vi "Keyboard Input with Sensitivity Support.vi"(0 "error in (no error)":errorcluster, 1 "Speed step":dbl, 2 "Previous Control Cluster":T2 {"Yaw Speed" scale=-1.0..1.0; "Vertical Speed" scale=-1.0..1.0; "Pitch" scale=-1.0..1.0; "Roll" scale=-1.0..1.0}, 3 "device ID":refnum<k1>) -> (4 "Control Cluster":T3 {"Roll" scale=-1.0..1.0; "Pitch" scale=-1.0..1.0; "Vertical Speed" scale=-1.0..1.0; "Yaw Speed" scale=-1.0..1.0}, 5 "error out":errorcluster, 6 "Buttons control":T1)   [LabVIEW 2014]
uses:
  <vilib>/Utility/inputDevices.llb/keyboardAcquire.vi
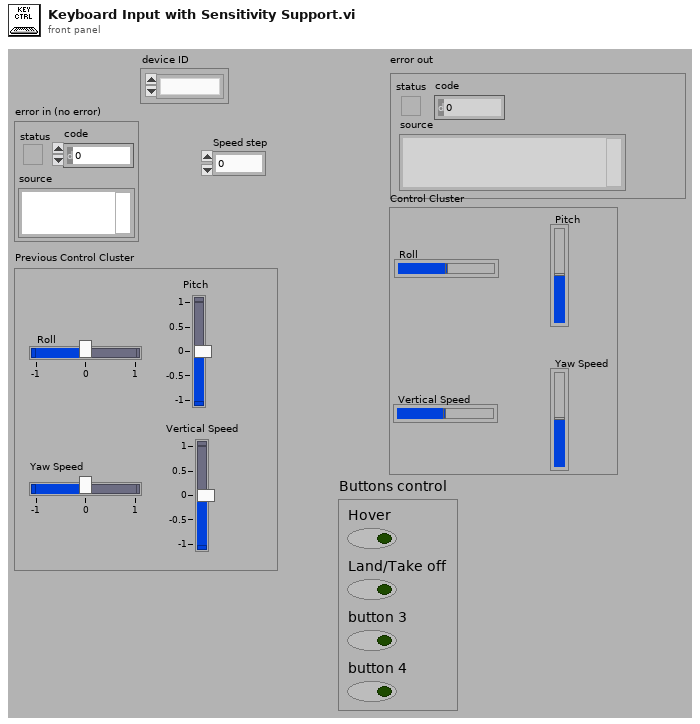
[diagram p1: front panel]
types:
  T1 = cluster{"Hover":bool, "Land/Take off":bool, "button 3":bool, "button 4":bool}
  T2 = cluster{"Roll":sgl, "Pitch":sgl, "Vertical Speed":sgl, "Yaw Speed":sgl}
  T3 = cluster{"Roll":dbl, "Pitch":dbl, "Vertical Speed":dbl, "Yaw Speed":dbl}
  T4 = enum16{"0", "1", "2", "3", "4", "5", "6", "7", "8", "9", "A", "B", "C", "D", "E", "F", "G", "H", "I", "J", "K", "L", "M", "N", "O", "P", "Q", "R", "S", "T", "U", "V", "W", "X", "Y", "Z", "F1", "F2", "F3", "F4", "F5", "F6", "F7", "F8", "F9", "F10", "F11", "F12", "F13", "F14", "F15", "ADD", "BACK", "BACKSLASH", "CAPITAL", "COMMA", "DECIMAL", "DELETE", "DIVIDE", "DOWN", "END", "EQUALS", "ESCAPE", "GRAVE (`)", "HOME", "INSERT", "LBRACKET", "LCONTROL", "LEFT", "L ALT", "LSHIFT", "LWIN", "MINUS", "MULTIPLY", "NEXT", "NUMLOCK", "NUMPAD_0", "NUMPAD_1", "NUMPAD_2", "NUMPAD_3", "NUMPAD_4", "NUMPAD_5", "NUMPAD_6", "NUMPAD_7", "NUMPAD_8", "NUMPAD_9", "PAUSE", "PERIOD", "PRIOR (PG UP)", "RBRACKET", "RCONTROL", "RETURN", "RIGHT", "R ALT", "RSHIFT", "RWIN", "SCROLL", "SEMICOLON", "SLASH", "SPACE", "SUBTRACT", "TAB", "UP", "ENTER (num pad)", "' (quote)"}[]
  T5 = enum16{"0", "1", "2", "3", "4", "5", "6", "7", "8", "9", "A", "B", "C", "D", "E", "F", "G", "H", "I", "J", "K", "L", "M", "N", "O", "P", "Q", "R", "S", "T", "U", "V", "W", "X", "Y", "Z", "F1", "F2", "F3", "F4", "F5", "F6", "F7", "F8", "F9", "F10", "F11", "F12", "F13", "F14", "F15", "ADD", "BACK", "BACKSLASH", "CAPITAL", "COMMA", "DECIMAL", "DELETE", "DIVIDE", "DOWN", "END", "EQUALS", "ESCAPE", "GRAVE (`)", "HOME", "INSERT", "LBRACKET", "LCONTROL", "LEFT", "L ALT", "LSHIFT", "LWIN", "MINUS", "MULTIPLY", "NEXT", "NUMLOCK", "NUMPAD_0", "NUMPAD_1", "NUMPAD_2", "NUMPAD_3", "NUMPAD_4", "NUMPAD_5", "NUMPAD_6", "NUMPAD_7", "NUMPAD_8", "NUMPAD_9", "PAUSE", "PERIOD", "PRIOR (PG UP)", "RBRACKET", "RCONTROL", "RETURN", "RIGHT", "R ALT", "RSHIFT", "RWIN", "SCROLL", "SEMICOLON", "SLASH", "SPACE", "SUBTRACT", "TAB", "UP", "ENTER (num pad)", "' (quote)"}
  T6 = cluster{dbl, dbl, "New Speed":dbl, "New Speed":dbl}
  T7 = cluster{dbl, "New Speed":dbl, "New Speed":dbl, dbl}
  T8 = cluster{"New Speed":dbl, dbl, "New Speed":dbl, dbl}
  T9 = cluster{dbl, "New Speed":dbl, dbl, "New Speed":dbl}
  T10 = cluster{"New Speed":dbl, dbl, dbl, "New Speed":dbl}
  T11 = cluster{"New Speed":dbl, "New Speed":dbl, dbl, dbl}
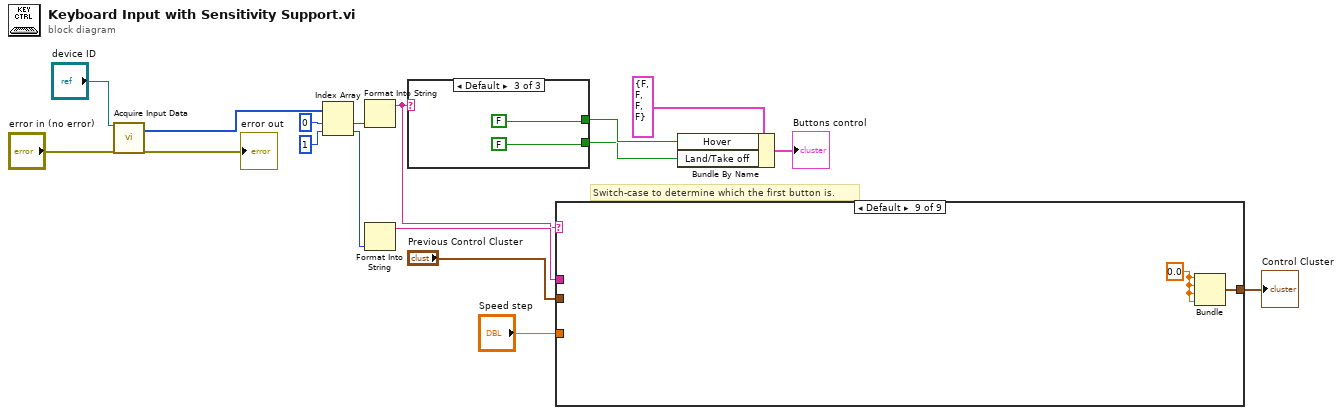
[diagram p0: block diagram]
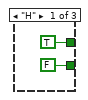
[diagram p2: hidden frame]
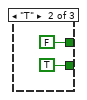
[diagram p3: hidden frame]
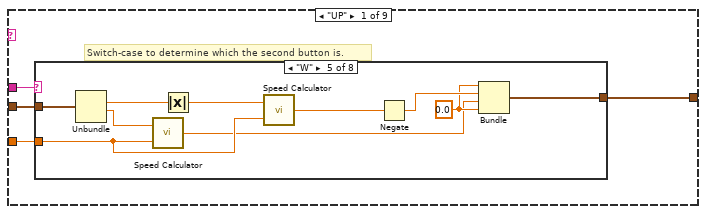
[diagram p4: hidden frame]
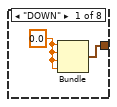
[diagram p5: hidden frame]
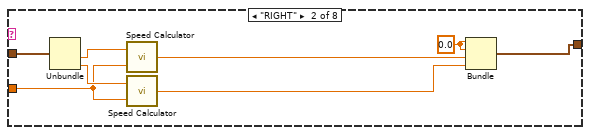
[diagram p6: hidden frame]
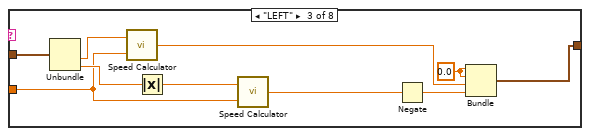
[diagram p7: hidden frame]
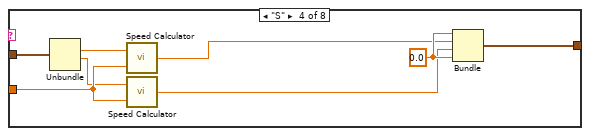
[diagram p8: hidden frame]
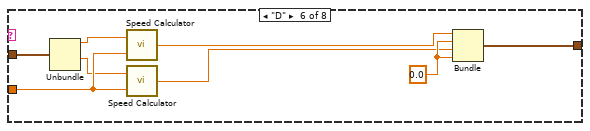
[diagram p9: hidden frame]
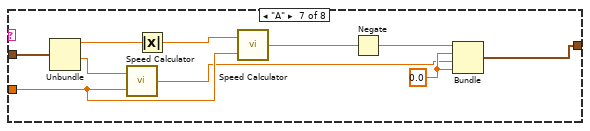
[diagram p10: hidden frame]
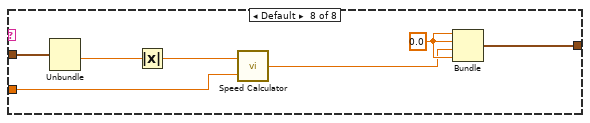
[diagram p11: hidden frame]
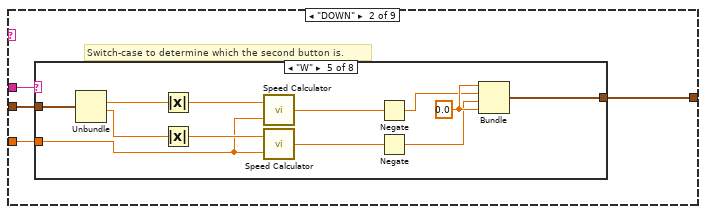
[diagram p12: hidden frame]
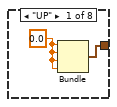
[diagram p13: hidden frame]
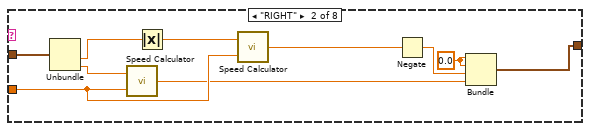
[diagram p14: hidden frame]
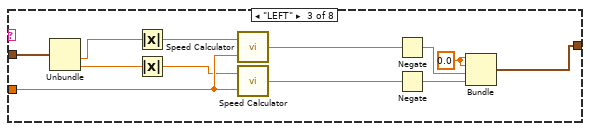
[diagram p15: hidden frame]
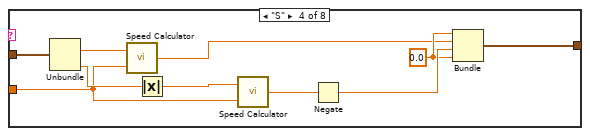
[diagram p16: hidden frame]
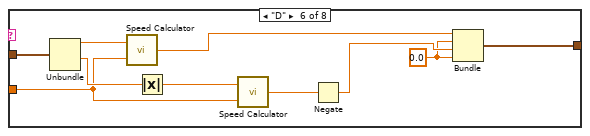
[diagram p17: hidden frame]
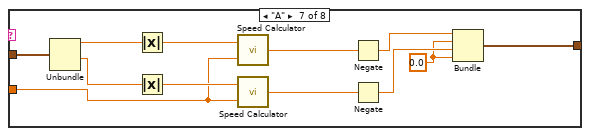
[diagram p18: hidden frame]
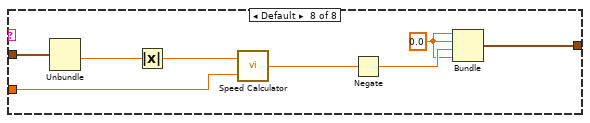
[diagram p19: hidden frame]
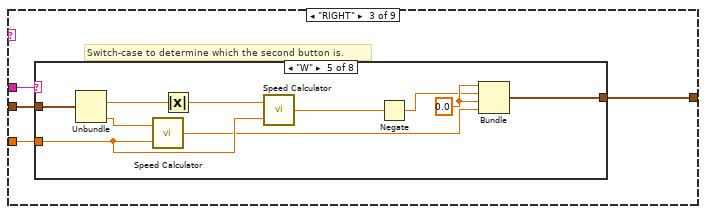
[diagram p20: hidden frame]
diagram:
  # "Switch-case to determine which the first button is."
  n1 = call-poly <vilib>:"Acquire Input Data.vi"("device ID"="device ID", "error in (no error)"="error in (no error)") -> ("keys pressed"=w12:T4, "error out"=→"error out":errorcluster)  [unwired: 15 in, 1 out]
  n2 = Index Array(array=w12, index #1=0, index #2=1) -> (element #1=w16:T5, element #2=w10:T5)
  n3 = Format Into String(w16) -> (resulting string=w5:string)  [unwired: 3 in, 1 out]
  n4 = Format Into String(w10) -> (resulting string=w9:string)  [unwired: 3 in, 1 out]
  n5 = case shown="Default" w5 {
    tunnel: [TRUE FALSE FALSE] -> w2
    tunnel: [FALSE TRUE FALSE] -> w1
    frame "H" {
    }
    frame "T" {
    }
    frame Default {
    }
  }
  n6 = case shown="Default" w5 {
    tunnel: w9 -> [w27 w93 w173 w240 w319 w385 w465 w531 _]
    tunnel: [w26 w92 w172 w238 w318 w384 w464 w530 w609] -> w7
    tunnel: "Speed step" -> [w25 w94 w174 w239 w320 w386 w466 w532 _]
    tunnel: "Previous Control Cluster" -> [w24 w91 w171 w237 w317 w383 w463 w529 _]
    frame "UP" {
      # "Switch-case to determine which the second button is."
      n7 = case shown="\"W\"" w27 {
        tunnel: [w28 w36 w47 w55 w65 w73 w83 w89] -> w26
        tunnel: w25 -> [_ w32 w41 w52 w59 w69 w78 w88]
        tunnel: w24 -> [_ w35 w44 w53 w62 w71 w80 w86]
        frame "DOWN" {
          w29 = 0.0
          n8 = Bundle(w29, w29, w29, w29) -> (w28:cluster{dbl, dbl, dbl, dbl})  [unwired: 1 in]
        }
        frame "RIGHT" {
          w37 = 0.0
          n9 = Unbundle(w35) -> ("Vertical Speed"=w30:sgl, "Yaw Speed"=w33:sgl)  [unwired: 2 out]
          n10 = call "Speed Calculator.vi"("Speed step"=w32, "Previous Speed"=w30) -> ("New Speed"=w34:dbl)
          n11 = call "Speed Calculator.vi"("Speed step"=w32, "Previous Speed"=w33) -> ("New Speed"=w31:dbl)
          n12 = Bundle(w37, w37, "New Speed"=w34, "New Speed"=w31) -> (w36:T6)  [unwired: 1 in]
        }
        frame "LEFT" {
          w45 = 0.0
          n13 = Unbundle(w44) -> ("Vertical Speed"=w40:sgl, "Yaw Speed"=w43:sgl)  [unwired: 2 out]
          n14 = call "Speed Calculator.vi"("Speed step"=w41, "Previous Speed"=w40) -> ("New Speed"=w39:dbl)
          n15 = Absolute Value(x=w43) -> (abs(x)=w42:sgl)
          n16 = call "Speed Calculator.vi"("Speed step"=w41, "Previous Speed"=w42) -> ("New Speed"=w38:dbl)
          n17 = Negate(x=w38) -> (-x=w46:dbl)
          n18 = Bundle(w45, w45, "New Speed"=w39, w46) -> (w47:cluster{dbl, dbl, "New Speed":dbl, dbl})  [unwired: 1 in]
        }
        frame "S" {
          w54 = 0.0
          n19 = Unbundle(w53) -> ("Pitch"=w48:sgl, "Vertical Speed"=w51:sgl)  [unwired: 2 out]
          n20 = call "Speed Calculator.vi"("Speed step"=w52, "Previous Speed"=w48) -> ("New Speed"=w49:dbl)
          n21 = call "Speed Calculator.vi"("Speed step"=w52, "Previous Speed"=w51) -> ("New Speed"=w50:dbl)
          n22 = Bundle(w54, "New Speed"=w49, "New Speed"=w50, w54) -> (w55:T7)  [unwired: 1 in]
        }
        frame "W" {
          w63 = 0.0
          n23 = Unbundle(w62) -> ("Pitch"=w61:sgl, "Vertical Speed"=w58:sgl)  [unwired: 2 out]
          n24 = call "Speed Calculator.vi"("Speed step"=w59, "Previous Speed"=w58) -> ("New Speed"=w57:dbl)
          n25 = Absolute Value(x=w61) -> (abs(x)=w60:sgl)
          n26 = call "Speed Calculator.vi"("Speed step"=w59, "Previous Speed"=w60) -> ("New Speed"=w56:dbl)
          n27 = Negate(x=w56) -> (-x=w64:dbl)
          n28 = Bundle(w63, w64, "New Speed"=w57, w63) -> (w65:cluster{dbl, dbl, "New Speed":dbl, dbl})  [unwired: 1 in]
        }
        frame "D" {
          w72 = 0.0
          n29 = Unbundle(w71) -> ("Roll"=w70:sgl, "Vertical Speed"=w68:sgl)  [unwired: 2 out]
          n30 = call "Speed Calculator.vi"("Speed step"=w69, "Previous Speed"=w70) -> ("New Speed"=w66:dbl)
          n31 = call "Speed Calculator.vi"("Speed step"=w69, "Previous Speed"=w68) -> ("New Speed"=w67:dbl)
          n32 = Bundle("New Speed"=w66, w72, "New Speed"=w67, w72) -> (w73:T8)  [unwired: 1 in]
        }
        frame "A" {
          w81 = 0.0
          n33 = Unbundle(w80) -> ("Roll"=w76:sgl, "Vertical Speed"=w79:sgl)  [unwired: 2 out]
          n34 = call "Speed Calculator.vi"("Speed step"=w78, "Previous Speed"=w79) -> ("New Speed"=w74:dbl)
          n35 = Absolute Value(x=w76) -> (abs(x)=w77:sgl)
          n36 = call "Speed Calculator.vi"("Speed step"=w78, "Previous Speed"=w77) -> ("New Speed"=w75:dbl)
          n37 = Negate(x=w75) -> (-x=w82:dbl)
          n38 = Bundle(w82, w81, "New Speed"=w74, w81) -> (w83:cluster{dbl, dbl, "New Speed":dbl, dbl})  [unwired: 1 in]
        }
        frame Default {
          w90 = 0.0
          n39 = Unbundle(w86) -> ("Vertical Speed"=w85:sgl)  [unwired: 3 out]
          n40 = Absolute Value(x=w85) -> (abs(x)=w84:sgl)
          n41 = call "Speed Calculator.vi"("Speed step"=w88, "Previous Speed"=w84) -> ("New Speed"=w87:dbl)
          n42 = Bundle(w90, w90, "New Speed"=w87, w90) -> (w89:cluster{dbl, dbl, "New Speed":dbl, dbl})  [unwired: 1 in]
        }
      }
    }
    frame "DOWN" {
      # "Switch-case to determine which the second button is."
      n43 = case shown="\"W\"" w93 {
        tunnel: [w96 w105 w118 w127 w140 w149 w162 w168] -> w92
        tunnel: w94 -> [_ w100 w113 w122 w133 w143 w151 w164]
        tunnel: w91 -> [_ w103 w116 w125 w138 w147 w158 w167]
        frame "UP" {
          w95 = 0.0
          n44 = Bundle(w95, w95, w95, w95) -> (w96:cluster{dbl, dbl, dbl, dbl})  [unwired: 1 in]
        }
        frame "RIGHT" {
          w104 = 0.0
          n45 = Unbundle(w103) -> ("Vertical Speed"=w102:sgl, "Yaw Speed"=w99:sgl)  [unwired: 2 out]
          n46 = call "Speed Calculator.vi"("Speed step"=w100, "Previous Speed"=w99) -> ("New Speed"=w98:dbl)
          n47 = Absolute Value(x=w102) -> (abs(x)=w101:sgl)
          n48 = call "Speed Calculator.vi"("Speed step"=w100, "Previous Speed"=w101) -> ("New Speed"=w97:dbl)
          n49 = Negate(x=w97) -> (-x=w106:dbl)
          n50 = Bundle(w104, w104, w106, "New Speed"=w98) -> (w105:cluster{dbl, dbl, dbl, "New Speed":dbl})  [unwired: 1 in]
        }
        frame "LEFT" {
          w117 = 0.0
          n51 = Unbundle(w116) -> ("Vertical Speed"=w115:sgl, "Yaw Speed"=w111:sgl)  [unwired: 2 out]
          n52 = Absolute Value(x=w115) -> (abs(x)=w114:sgl)
          n53 = Absolute Value(x=w111) -> (abs(x)=w112:sgl)
          n54 = call "Speed Calculator.vi"("Speed step"=w113, "Previous Speed"=w114) -> ("New Speed"=w110:dbl)
          n55 = call "Speed Calculator.vi"("Speed step"=w113, "Previous Speed"=w112) -> ("New Speed"=w109:dbl)
          n56 = Negate(x=w110) -> (-x=w108:dbl)
          n57 = Negate(x=w109) -> (-x=w107:dbl)
          n58 = Bundle(w117, w117, w108, w107) -> (w118:cluster{dbl, dbl, dbl, dbl})  [unwired: 1 in]
        }
        frame "S" {
          w126 = 0.0
          n59 = Unbundle(w125) -> ("Pitch"=w121:sgl, "Yaw Speed"=w124:sgl)  [unwired: 2 out]
          n60 = call "Speed Calculator.vi"("Speed step"=w122, "Previous Speed"=w121) -> ("New Speed"=w120:dbl)
          n61 = Absolute Value(x=w124) -> (abs(x)=w123:sgl)
          n62 = call "Speed Calculator.vi"("Speed step"=w122, "Previous Speed"=w123) -> ("New Speed"=w119:dbl)
          n63 = Negate(x=w119) -> (-x=w128:dbl)
          n64 = Bundle(w126, "New Speed"=w120, w128, w126) -> (w127:cluster{dbl, "New Speed":dbl, dbl, dbl})  [unwired: 1 in]
        }
        frame "W" {
          w139 = 0.0
          n65 = Unbundle(w138) -> ("Pitch"=w137:sgl, "Vertical Speed"=w135:sgl)  [unwired: 2 out]
          n66 = Absolute Value(x=w137) -> (abs(x)=w136:sgl)
          n67 = Absolute Value(x=w135) -> (abs(x)=w134:sgl)
          n68 = call "Speed Calculator.vi"("Speed step"=w133, "Previous Speed"=w136) -> ("New Speed"=w132:dbl)
          n69 = call "Speed Calculator.vi"("Speed step"=w133, "Previous Speed"=w134) -> ("New Speed"=w131:dbl)
          n70 = Negate(x=w132) -> (-x=w130:dbl)
          n71 = Negate(x=w131) -> (-x=w129:dbl)
          n72 = Bundle(w139, w130, w129, w139) -> (w140:cluster{dbl, dbl, dbl, dbl})  [unwired: 1 in]
        }
        frame "D" {
          w148 = 0.0
          n73 = Unbundle(w147) -> ("Roll"=w141:sgl, "Vertical Speed"=w146:sgl)  [unwired: 2 out]
          n74 = call "Speed Calculator.vi"("Speed step"=w143, "Previous Speed"=w141) -> ("New Speed"=w142:dbl)
          n75 = Absolute Value(x=w146) -> (abs(x)=w145:sgl)
          n76 = call "Speed Calculator.vi"("Speed step"=w143, "Previous Speed"=w145) -> ("New Speed"=w144:dbl)
          n77 = Negate(x=w144) -> (-x=w150:dbl)
          n78 = Bundle("New Speed"=w142, w148, w150, w148) -> (w149:cluster{"New Speed":dbl, dbl, dbl, dbl})  [unwired: 1 in]
        }
        frame "A" {
          w160 = 0.0
          n79 = Unbundle(w158) -> ("Roll"=w157:sgl, "Vertical Speed"=w155:sgl)  [unwired: 2 out]
          n80 = Absolute Value(x=w157) -> (abs(x)=w156:sgl)
          n81 = Absolute Value(x=w155) -> (abs(x)=w154:sgl)
          n82 = call "Speed Calculator.vi"("Speed step"=w151, "Previous Speed"=w156) -> ("New Speed"=w152:dbl)
          n83 = call "Speed Calculator.vi"("Speed step"=w151, "Previous Speed"=w154) -> ("New Speed"=w153:dbl)
          n84 = Negate(x=w152) -> (-x=w159:dbl)
          n85 = Negate(x=w153) -> (-x=w161:dbl)
          n86 = Bundle(w159, w160, w161, w160) -> (w162:cluster{dbl, dbl, dbl, dbl})  [unwired: 1 in]
        }
        frame Default {
          w169 = 0.0
          n87 = Unbundle(w167) -> ("Vertical Speed"=w163:sgl)  [unwired: 3 out]
          n88 = Absolute Value(x=w163) -> (abs(x)=w166:sgl)
          n89 = call "Speed Calculator.vi"("Speed step"=w164, "Previous Speed"=w166) -> ("New Speed"=w165:dbl)
          n90 = Negate(x=w165) -> (-x=w170:dbl)
          n91 = Bundle(w169, w169, w170, w169) -> (w168:cluster{dbl, dbl, dbl, dbl})  [unwired: 1 in]
        }
      }
    }
    frame "RIGHT" {
      # "Switch-case to determine which the second button is."
      n92 = case shown="\"W\"" w173 {
        tunnel: [w181 w190 w193 w202 w212 w220 w230 w235] -> w172
        tunnel: w174 -> [w177 w185 _ w197 w205 w215 w221 w231]
        tunnel: w171 -> [w180 w189 _ w200 w209 w218 w227 w234]
        frame "UP" {
          w182 = 0.0
          n93 = Unbundle(w180) -> ("Vertical Speed"=w179:sgl, "Yaw Speed"=w178:sgl)  [unwired: 2 out]
          n94 = call "Speed Calculator.vi"("Speed step"=w177, "Previous Speed"=w179) -> ("New Speed"=w176:dbl)
          n95 = call "Speed Calculator.vi"("Speed step"=w177, "Previous Speed"=w178) -> ("New Speed"=w175:dbl)
          n96 = Bundle(w182, w182, "New Speed"=w176, "New Speed"=w175) -> (w181:T6)  [unwired: 1 in]
        }
        frame "DOWN" {
          w191 = 0.0
          n97 = Unbundle(w189) -> ("Vertical Speed"=w188:sgl, "Yaw Speed"=w184:sgl)  [unwired: 2 out]
          n98 = call "Speed Calculator.vi"("Speed step"=w185, "Previous Speed"=w184) -> ("New Speed"=w183:dbl)
          n99 = Absolute Value(x=w188) -> (abs(x)=w187:sgl)
          n100 = call "Speed Calculator.vi"("Speed step"=w185, "Previous Speed"=w187) -> ("New Speed"=w186:dbl)
          n101 = Negate(x=w186) -> (-x=w192:dbl)
          n102 = Bundle(w191, w191, w192, "New Speed"=w183) -> (w190:cluster{dbl, dbl, dbl, "New Speed":dbl})  [unwired: 1 in]
        }
        frame "LEFT" {
          w194 = 0.0
          n103 = Bundle(w194, w194, w194, w194) -> (w193:cluster{dbl, dbl, dbl, dbl})  [unwired: 1 in]
        }
        frame "S" {
          w201 = 0.0
          n104 = Unbundle(w200) -> ("Pitch"=w199:sgl, "Yaw Speed"=w198:sgl)  [unwired: 2 out]
          n105 = call "Speed Calculator.vi"("Speed step"=w197, "Previous Speed"=w199) -> ("New Speed"=w196:dbl)
          n106 = call "Speed Calculator.vi"("Speed step"=w197, "Previous Speed"=w198) -> ("New Speed"=w195:dbl)
          n107 = Bundle(w201, "New Speed"=w196, w201, "New Speed"=w195) -> (w202:T9)  [unwired: 1 in]
        }
        frame "W" {
          w211 = 0.0
          n108 = Unbundle(w209) -> ("Pitch"=w208:sgl, "Yaw Speed"=w204:sgl)  [unwired: 2 out]
          n109 = call "Speed Calculator.vi"("Speed step"=w205, "Previous Speed"=w204) -> ("New Speed"=w203:dbl)
          n110 = Absolute Value(x=w208) -> (abs(x)=w207:sgl)
          n111 = call "Speed Calculator.vi"("Speed step"=w205, "Previous Speed"=w207) -> ("New Speed"=w206:dbl)
          n112 = Negate(x=w206) -> (-x=w210:dbl)
          n113 = Bundle(w211, w210, w211, "New Speed"=w203) -> (w212:cluster{dbl, dbl, dbl, "New Speed":dbl})  [unwired: 1 in]
        }
        frame "D" {
          w219 = 0.0
          n114 = Unbundle(w218) -> ("Roll"=w217:sgl, "Yaw Speed"=w216:sgl)  [unwired: 2 out]
          n115 = call "Speed Calculator.vi"("Speed step"=w215, "Previous Speed"=w217) -> ("New Speed"=w214:dbl)
          n116 = call "Speed Calculator.vi"("Speed step"=w215, "Previous Speed"=w216) -> ("New Speed"=w213:dbl)
          n117 = Bundle("New Speed"=w214, w219, w219, "New Speed"=w213) -> (w220:T10)  [unwired: 1 in]
        }
        frame "A" {
          w228 = 0.0
          n118 = Unbundle(w227) -> ("Roll"=w226:sgl, "Yaw Speed"=w223:sgl)  [unwired: 2 out]
          n119 = call "Speed Calculator.vi"("Speed step"=w221, "Previous Speed"=w223) -> ("New Speed"=w222:dbl)
          n120 = Absolute Value(x=w226) -> (abs(x)=w225:sgl)
          n121 = call "Speed Calculator.vi"("Speed step"=w221, "Previous Speed"=w225) -> ("New Speed"=w224:dbl)
          n122 = Negate(x=w224) -> (-x=w229:dbl)
          n123 = Bundle(w229, w228, w228, "New Speed"=w222) -> (w230:cluster{dbl, dbl, dbl, "New Speed":dbl})  [unwired: 1 in]
        }
        frame Default {
          w236 = 0.0
          n124 = Unbundle(w234) -> ("Yaw Speed"=w233:sgl)  [unwired: 3 out]
          n125 = call "Speed Calculator.vi"("Speed step"=w231, "Previous Speed"=w233) -> ("New Speed"=w232:dbl)
          n126 = Bundle(w236, w236, w236, "New Speed"=w232) -> (w235:cluster{dbl, dbl, dbl, "New Speed":dbl})  [unwired: 1 in]
        }
      }
    }
    frame "LEFT" {
      # "Switch-case to determine which the second button is."
      n127 = case shown="\"W\"" w240 {
        tunnel: [w248 w260 w263 w273 w286 w295 w308 w316] -> w238
        tunnel: w239 -> [w241 w251 _ w265 w275 w287 w301 w309]
        tunnel: w237 -> [w247 w259 _ w271 w284 w293 w306 w313]
        frame "UP" {
          w249 = 0.0
          n128 = Unbundle(w247) -> ("Vertical Speed"=w242:sgl, "Yaw Speed"=w246:sgl)  [unwired: 2 out]
          n129 = call "Speed Calculator.vi"("Speed step"=w241, "Previous Speed"=w242) -> ("New Speed"=w243:dbl)
          n130 = Absolute Value(x=w246) -> (abs(x)=w245:sgl)
          n131 = call "Speed Calculator.vi"("Speed step"=w241, "Previous Speed"=w245) -> ("New Speed"=w244:dbl)
          n132 = Negate(x=w244) -> (-x=w250:dbl)
          n133 = Bundle(w249, w249, "New Speed"=w243, w250) -> (w248:cluster{dbl, dbl, "New Speed":dbl, dbl})  [unwired: 1 in]
        }
        frame "DOWN" {
          w261 = 0.0
          n134 = Unbundle(w259) -> ("Vertical Speed"=w253:sgl, "Yaw Speed"=w252:sgl)  [unwired: 2 out]
          n135 = Absolute Value(x=w253) -> (abs(x)=w255:sgl)
          n136 = Absolute Value(x=w252) -> (abs(x)=w254:sgl)
          n137 = call "Speed Calculator.vi"("Speed step"=w251, "Previous Speed"=w255) -> ("New Speed"=w257:dbl)
          n138 = call "Speed Calculator.vi"("Speed step"=w251, "Previous Speed"=w254) -> ("New Speed"=w256:dbl)
          n139 = Negate(x=w257) -> (-x=w258:dbl)
          n140 = Negate(x=w256) -> (-x=w262:dbl)
          n141 = Bundle(w261, w261, w258, w262) -> (w260:cluster{dbl, dbl, dbl, dbl})  [unwired: 1 in]
        }
        frame "RIGHT" {
          w264 = 0.0
          n142 = Bundle(w264, w264, w264, w264) -> (w263:cluster{dbl, dbl, dbl, dbl})  [unwired: 1 in]
        }
        frame "S" {
          w272 = 0.0
          n143 = Unbundle(w271) -> ("Pitch"=w270:sgl, "Yaw Speed"=w268:sgl)  [unwired: 2 out]
          n144 = call "Speed Calculator.vi"("Speed step"=w265, "Previous Speed"=w270) -> ("New Speed"=w269:dbl)
          n145 = Absolute Value(x=w268) -> (abs(x)=w267:sgl)
          n146 = call "Speed Calculator.vi"("Speed step"=w265, "Previous Speed"=w267) -> ("New Speed"=w266:dbl)
          n147 = Negate(x=w266) -> (-x=w274:dbl)
          n148 = Bundle(w272, "New Speed"=w269, w272, w274) -> (w273:cluster{dbl, "New Speed":dbl, dbl, dbl})  [unwired: 1 in]
        }
        frame "W" {
          w285 = 0.0
          n149 = Unbundle(w284) -> ("Pitch"=w283:sgl, "Yaw Speed"=w282:sgl)  [unwired: 2 out]
          n150 = Absolute Value(x=w283) -> (abs(x)=w280:sgl)
          n151 = Absolute Value(x=w282) -> (abs(x)=w281:sgl)
          n152 = call "Speed Calculator.vi"("Speed step"=w275, "Previous Speed"=w280) -> ("New Speed"=w279:dbl)
          n153 = call "Speed Calculator.vi"("Speed step"=w275, "Previous Speed"=w281) -> ("New Speed"=w278:dbl)
          n154 = Negate(x=w279) -> (-x=w277:dbl)
          n155 = Negate(x=w278) -> (-x=w276:dbl)
          n156 = Bundle(w285, w277, w285, w276) -> (w286:cluster{dbl, dbl, dbl, dbl})  [unwired: 1 in]
        }
        frame "D" {
          w294 = 0.0
          n157 = Unbundle(w293) -> ("Roll"=w292:sgl, "Yaw Speed"=w290:sgl)  [unwired: 2 out]
          n158 = call "Speed Calculator.vi"("Speed step"=w287, "Previous Speed"=w292) -> ("New Speed"=w291:dbl)
          n159 = Absolute Value(x=w290) -> (abs(x)=w289:sgl)
          n160 = call "Speed Calculator.vi"("Speed step"=w287, "Previous Speed"=w289) -> ("New Speed"=w288:dbl)
          n161 = Negate(x=w288) -> (-x=w296:dbl)
          n162 = Bundle("New Speed"=w291, w294, w294, w296) -> (w295:cluster{"New Speed":dbl, dbl, dbl, dbl})  [unwired: 1 in]
        }
        frame "A" {
          w307 = 0.0
          n163 = Unbundle(w306) -> ("Roll"=w305:sgl, "Yaw Speed"=w304:sgl)  [unwired: 2 out]
          n164 = Absolute Value(x=w305) -> (abs(x)=w303:sgl)
          n165 = Absolute Value(x=w304) -> (abs(x)=w302:sgl)
          n166 = call "Speed Calculator.vi"("Speed step"=w301, "Previous Speed"=w303) -> ("New Speed"=w300:dbl)
          n167 = call "Speed Calculator.vi"("Speed step"=w301, "Previous Speed"=w302) -> ("New Speed"=w299:dbl)
          n168 = Negate(x=w300) -> (-x=w298:dbl)
          n169 = Negate(x=w299) -> (-x=w297:dbl)
          n170 = Bundle(w298, w307, w307, w297) -> (w308:cluster{dbl, dbl, dbl, dbl})  [unwired: 1 in]
        }
        frame Default {
          w315 = 0.0
          n171 = Unbundle(w313) -> ("Yaw Speed"=w312:sgl)  [unwired: 3 out]
          n172 = Absolute Value(x=w312) -> (abs(x)=w311:sgl)
          n173 = call "Speed Calculator.vi"("Speed step"=w309, "Previous Speed"=w311) -> ("New Speed"=w310:dbl)
          n174 = Negate(x=w310) -> (-x=w314:dbl)
          n175 = Bundle(w315, w315, w315, w314) -> (w316:cluster{dbl, dbl, dbl, dbl})  [unwired: 1 in]
        }
      }
    }
    frame "S" {
      # "Switch-case to determine which the second button is."
      n176 = case shown="\"W\"" w319 {
        tunnel: [w328 w337 w346 w355 w357 w365 w375 w382] -> w318
        tunnel: w320 -> [w321 w329 w339 w347 _ w359 w367 w377]
        tunnel: w317 -> [w327 w335 w345 w354 _ w364 w373 w380]
        frame "UP" {
          w326 = 0.0
          n177 = Unbundle(w327) -> ("Pitch"=w325:sgl, "Vertical Speed"=w324:sgl)  [unwired: 2 out]
          n178 = call "Speed Calculator.vi"("Speed step"=w321, "Previous Speed"=w325) -> ("New Speed"=w323:dbl)
          n179 = call "Speed Calculator.vi"("Speed step"=w321, "Previous Speed"=w324) -> ("New Speed"=w322:dbl)
          n180 = Bundle(w326, "New Speed"=w323, "New Speed"=w322, w326) -> (w328:T7)  [unwired: 1 in]
        }
        frame "DOWN" {
          w336 = 0.0
          n181 = Unbundle(w335) -> ("Pitch"=w334:sgl, "Vertical Speed"=w333:sgl)  [unwired: 2 out]
          n182 = call "Speed Calculator.vi"("Speed step"=w329, "Previous Speed"=w334) -> ("New Speed"=w330:dbl)
          n183 = Absolute Value(x=w333) -> (abs(x)=w332:sgl)
          n184 = call "Speed Calculator.vi"("Speed step"=w329, "Previous Speed"=w332) -> ("New Speed"=w331:dbl)
          n185 = Negate(x=w331) -> (-x=w338:dbl)
          n186 = Bundle(w336, "New Speed"=w330, w338, w336) -> (w337:cluster{dbl, "New Speed":dbl, dbl, dbl})  [unwired: 1 in]
        }
        frame "RIGHT" {
          w344 = 0.0
          n187 = Unbundle(w345) -> ("Pitch"=w343:sgl, "Vertical Speed"=w340:sgl)  [unwired: 2 out]
          n188 = call "Speed Calculator.vi"("Speed step"=w339, "Previous Speed"=w343) -> ("New Speed"=w342:dbl)
          n189 = call "Speed Calculator.vi"("Speed step"=w339, "Previous Speed"=w340) -> ("New Speed"=w341:dbl)
          n190 = Bundle(w344, "New Speed"=w342, w344, "New Speed"=w341) -> (w346:T9)  [unwired: 1 in]
        }
        frame "LEFT" {
          w353 = 0.0
          n191 = Unbundle(w354) -> ("Pitch"=w348:sgl, "Yaw Speed"=w352:sgl)  [unwired: 2 out]
          n192 = call "Speed Calculator.vi"("Speed step"=w347, "Previous Speed"=w348) -> ("New Speed"=w349:dbl)
          n193 = Absolute Value(x=w352) -> (abs(x)=w351:sgl)
          n194 = call "Speed Calculator.vi"("Speed step"=w347, "Previous Speed"=w351) -> ("New Speed"=w350:dbl)
          n195 = Negate(x=w350) -> (-x=w356:dbl)
          n196 = Bundle(w353, "New Speed"=w349, w353, w356) -> (w355:cluster{dbl, "New Speed":dbl, dbl, dbl})  [unwired: 1 in]
        }
        frame "W" {
          w358 = 0.0
          n197 = Bundle(w358, w358, w358, w358) -> (w357:cluster{dbl, dbl, dbl, dbl})  [unwired: 1 in]
        }
        frame "D" {
          w366 = 0.0
          n198 = Unbundle(w364) -> ("Roll"=w363:sgl, "Pitch"=w361:sgl)  [unwired: 2 out]
          n199 = call "Speed Calculator.vi"("Speed step"=w359, "Previous Speed"=w363) -> ("New Speed"=w362:dbl)
          n200 = call "Speed Calculator.vi"("Speed step"=w359, "Previous Speed"=w361) -> ("New Speed"=w360:dbl)
          n201 = Bundle("New Speed"=w362, "New Speed"=w360, w366, w366) -> (w365:T11)  [unwired: 1 in]
        }
        frame "A" {
          w376 = 0.0
          n202 = Unbundle(w373) -> ("Roll"=w372:sgl, "Pitch"=w369:sgl)  [unwired: 2 out]
          n203 = call "Speed Calculator.vi"("Speed step"=w367, "Previous Speed"=w369) -> ("New Speed"=w368:dbl)
          n204 = Absolute Value(x=w372) -> (abs(x)=w371:sgl)
          n205 = call "Speed Calculator.vi"("Speed step"=w367, "Previous Speed"=w371) -> ("New Speed"=w370:dbl)
          n206 = Negate(x=w370) -> (-x=w374:dbl)
          n207 = Bundle(w374, "New Speed"=w368, w376, w376) -> (w375:cluster{dbl, "New Speed":dbl, dbl, dbl})  [unwired: 1 in]
        }
        frame Default {
          w381 = 0.0
          n208 = Unbundle(w380) -> ("Pitch"=w379:sgl)  [unwired: 3 out]
          n209 = call "Speed Calculator.vi"("Speed step"=w377, "Previous Speed"=w379) -> ("New Speed"=w378:dbl)
          n210 = Bundle(w381, "New Speed"=w378, w381, w381) -> (w382:cluster{dbl, "New Speed":dbl, dbl, dbl})  [unwired: 1 in]
        }
      }
    }
    frame "W" {
      # "Switch-case to determine which the second button is."
      n211 = case shown="\"S\"" w385 {
        tunnel: [w396 w407 w418 w430 w431 w441 w452 w462] -> w384
        tunnel: w386 -> [w391 w399 w411 w421 _ w435 w443 w456]
        tunnel: w383 -> [w395 w406 w417 w426 _ w439 w446 w459]
        frame "UP" {
          w387 = 0.0
          n212 = Unbundle(w395) -> ("Roll"=w394:sgl, "Vertical Speed"=w390:sgl)  [unwired: 2 out]
          n213 = call "Speed Calculator.vi"("Speed step"=w391, "Previous Speed"=w390) -> ("New Speed"=w389:dbl)
          n214 = Absolute Value(x=w394) -> (abs(x)=w393:sgl)
          n215 = call "Speed Calculator.vi"("Speed step"=w391, "Previous Speed"=w393) -> ("New Speed"=w392:dbl)
          n216 = Negate(x=w392) -> (-x=w388:dbl)
          n217 = Bundle(w387, w388, "New Speed"=w389, w387) -> (w396:cluster{dbl, dbl, "New Speed":dbl, dbl})  [unwired: 1 in]
        }
        frame "DOWN" {
          w398 = 0.0
          n218 = Unbundle(w406) -> ("Roll"=w405:sgl, "Vertical Speed"=w401:sgl)  [unwired: 2 out]
          n219 = Absolute Value(x=w405) -> (abs(x)=w404:sgl)
          n220 = Absolute Value(x=w401) -> (abs(x)=w402:sgl)
          n221 = call "Speed Calculator.vi"("Speed step"=w399, "Previous Speed"=w404) -> ("New Speed"=w403:dbl)
          n222 = call "Speed Calculator.vi"("Speed step"=w399, "Previous Speed"=w402) -> ("New Speed"=w400:dbl)
          n223 = Negate(x=w403) -> (-x=w397:dbl)
          n224 = Negate(x=w400) -> (-x=w408:dbl)
          n225 = Bundle(w398, w397, w408, w398) -> (w407:cluster{dbl, dbl, dbl, dbl})  [unwired: 1 in]
        }
        frame "RIGHT" {
          w410 = 0.0
          n226 = Unbundle(w417) -> ("Roll"=w416:sgl, "Yaw Speed"=w414:sgl)  [unwired: 2 out]
          n227 = call "Speed Calculator.vi"("Speed step"=w411, "Previous Speed"=w414) -> ("New Speed"=w413:dbl)
          n228 = Absolute Value(x=w416) -> (abs(x)=w415:sgl)
          n229 = call "Speed Calculator.vi"("Speed step"=w411, "Previous Speed"=w415) -> ("New Speed"=w412:dbl)
          n230 = Negate(x=w412) -> (-x=w409:dbl)
          n231 = Bundle(w410, w409, w410, "New Speed"=w413) -> (w418:cluster{dbl, dbl, dbl, "New Speed":dbl})  [unwired: 1 in]
        }
        frame "LEFT" {
          w419 = 0.0
          n232 = Unbundle(w426) -> ("Roll"=w425:sgl, "Yaw Speed"=w423:sgl)  [unwired: 2 out]
          n233 = Absolute Value(x=w425) -> (abs(x)=w424:sgl)
          n234 = Absolute Value(x=w423) -> (abs(x)=w422:sgl)
          n235 = call "Speed Calculator.vi"("Speed step"=w421, "Previous Speed"=w424) -> ("New Speed"=w428:dbl)
          n236 = call "Speed Calculator.vi"("Speed step"=w421, "Previous Speed"=w422) -> ("New Speed"=w427:dbl)
          n237 = Negate(x=w428) -> (-x=w420:dbl)
          n238 = Negate(x=w427) -> (-x=w429:dbl)
          n239 = Bundle(w419, w420, w419, w429) -> (w430:cluster{dbl, dbl, dbl, dbl})  [unwired: 1 in]
        }
        frame "S" {
          w432 = 0.0
          n240 = Bundle(w432, w432, w432, w432) -> (w431:cluster{dbl, dbl, dbl, dbl})  [unwired: 1 in]
        }
        frame "D" {
          w442 = 0.0
          n241 = Unbundle(w439) -> ("Roll"=w434:sgl, "Pitch"=w438:sgl)  [unwired: 2 out]
          n242 = call "Speed Calculator.vi"("Speed step"=w435, "Previous Speed"=w434) -> ("New Speed"=w433:dbl)
          n243 = Absolute Value(x=w438) -> (abs(x)=w437:sgl)
          n244 = call "Speed Calculator.vi"("Speed step"=w435, "Previous Speed"=w437) -> ("New Speed"=w436:dbl)
          n245 = Negate(x=w436) -> (-x=w440:dbl)
          n246 = Bundle("New Speed"=w433, w440, w442, w442) -> (w441:cluster{"New Speed":dbl, dbl, dbl, dbl})  [unwired: 1 in]
        }
        frame "A" {
          w453 = 0.0
          n247 = Unbundle(w446) -> ("Roll"=w445:sgl, "Pitch"=w444:sgl)  [unwired: 2 out]
          n248 = Absolute Value(x=w445) -> (abs(x)=w448:sgl)
          n249 = Absolute Value(x=w444) -> (abs(x)=w447:sgl)
          n250 = call "Speed Calculator.vi"("Speed step"=w443, "Previous Speed"=w448) -> ("New Speed"=w450:dbl)
          n251 = call "Speed Calculator.vi"("Speed step"=w443, "Previous Speed"=w447) -> ("New Speed"=w449:dbl)
          n252 = Negate(x=w450) -> (-x=w451:dbl)
          n253 = Negate(x=w449) -> (-x=w454:dbl)
          n254 = Bundle(w451, w454, w453, w453) -> (w452:cluster{dbl, dbl, dbl, dbl})  [unwired: 1 in]
        }
        frame Default {
          w460 = 0.0
          n255 = Unbundle(w459) -> ("Pitch"=w455:sgl)  [unwired: 3 out]
          n256 = Absolute Value(x=w455) -> (abs(x)=w458:sgl)
          n257 = call "Speed Calculator.vi"("Speed step"=w456, "Previous Speed"=w458) -> ("New Speed"=w457:dbl)
          n258 = Negate(x=w457) -> (-x=w461:dbl)
          n259 = Bundle(w460, w461, w460, w460) -> (w462:cluster{dbl, dbl, dbl, dbl})  [unwired: 1 in]
        }
      }
    }
    frame "D" {
      # "Switch-case to determine which the second button is."
      n260 = case shown="\"W\"" w465 {
        tunnel: [w474 w483 w492 w501 w509 w519 w521 w528] -> w464
        tunnel: w466 -> [w468 w475 w485 w493 w503 w511 _ w523]
        tunnel: w463 -> [w472 w481 w490 w499 w508 w517 _ w526]
        frame "UP" {
          w473 = 0.0
          n261 = Unbundle(w472) -> ("Roll"=w471:sgl, "Vertical Speed"=w467:sgl)  [unwired: 2 out]
          n262 = call "Speed Calculator.vi"("Speed step"=w468, "Previous Speed"=w471) -> ("New Speed"=w470:dbl)
          n263 = call "Speed Calculator.vi"("Speed step"=w468, "Previous Speed"=w467) -> ("New Speed"=w469:dbl)
          n264 = Bundle("New Speed"=w470, w473, "New Speed"=w469, w473) -> (w474:T8)  [unwired: 1 in]
        }
        frame "DOWN" {
          w482 = 0.0
          n265 = Unbundle(w481) -> ("Roll"=w477:sgl, "Vertical Speed"=w480:sgl)  [unwired: 2 out]
          n266 = call "Speed Calculator.vi"("Speed step"=w475, "Previous Speed"=w477) -> ("New Speed"=w476:dbl)
          n267 = Absolute Value(x=w480) -> (abs(x)=w479:sgl)
          n268 = call "Speed Calculator.vi"("Speed step"=w475, "Previous Speed"=w479) -> ("New Speed"=w478:dbl)
          n269 = Negate(x=w478) -> (-x=w484:dbl)
          n270 = Bundle("New Speed"=w476, w482, w484, w482) -> (w483:cluster{"New Speed":dbl, dbl, dbl, dbl})  [unwired: 1 in]
        }
        frame "RIGHT" {
          w491 = 0.0
          n271 = Unbundle(w490) -> ("Roll"=w489:sgl, "Yaw Speed"=w488:sgl)  [unwired: 2 out]
          n272 = call "Speed Calculator.vi"("Speed step"=w485, "Previous Speed"=w489) -> ("New Speed"=w487:dbl)
          n273 = call "Speed Calculator.vi"("Speed step"=w485, "Previous Speed"=w488) -> ("New Speed"=w486:dbl)
          n274 = Bundle("New Speed"=w487, w491, w491, "New Speed"=w486) -> (w492:T10)  [unwired: 1 in]
        }
        frame "LEFT" {
          w500 = 0.0
          n275 = Unbundle(w499) -> ("Roll"=w495:sgl, "Yaw Speed"=w498:sgl)  [unwired: 2 out]
          n276 = call "Speed Calculator.vi"("Speed step"=w493, "Previous Speed"=w495) -> ("New Speed"=w494:dbl)
          n277 = Absolute Value(x=w498) -> (abs(x)=w497:sgl)
          n278 = call "Speed Calculator.vi"("Speed step"=w493, "Previous Speed"=w497) -> ("New Speed"=w496:dbl)
          n279 = Negate(x=w496) -> (-x=w502:dbl)
          n280 = Bundle("New Speed"=w494, w500, w500, w502) -> (w501:cluster{"New Speed":dbl, dbl, dbl, dbl})  [unwired: 1 in]
        }
        frame "S" {
          w510 = 0.0
          n281 = Unbundle(w508) -> ("Roll"=w507:sgl, "Pitch"=w506:sgl)  [unwired: 2 out]
          n282 = call "Speed Calculator.vi"("Speed step"=w503, "Previous Speed"=w507) -> ("New Speed"=w505:dbl)
          n283 = call "Speed Calculator.vi"("Speed step"=w503, "Previous Speed"=w506) -> ("New Speed"=w504:dbl)
          n284 = Bundle("New Speed"=w505, "New Speed"=w504, w510, w510) -> (w509:T11)  [unwired: 1 in]
        }
        frame "W" {
          w520 = 0.0
          n285 = Unbundle(w517) -> ("Roll"=w512:sgl, "Pitch"=w516:sgl)  [unwired: 2 out]
          n286 = call "Speed Calculator.vi"("Speed step"=w511, "Previous Speed"=w512) -> ("New Speed"=w513:dbl)
          n287 = Absolute Value(x=w516) -> (abs(x)=w515:sgl)
          n288 = call "Speed Calculator.vi"("Speed step"=w511, "Previous Speed"=w515) -> ("New Speed"=w514:dbl)
          n289 = Negate(x=w514) -> (-x=w518:dbl)
          n290 = Bundle("New Speed"=w513, w518, w520, w520) -> (w519:cluster{"New Speed":dbl, dbl, dbl, dbl})  [unwired: 1 in]
        }
        frame "A" {
          w522 = 0.0
          n291 = Bundle(w522, w522, w522, w522) -> (w521:cluster{dbl, dbl, dbl, dbl})  [unwired: 1 in]
        }
        frame Default {
          w527 = 0.0
          n292 = Unbundle(w526) -> ("Roll"=w525:sgl)  [unwired: 3 out]
          n293 = call "Speed Calculator.vi"("Speed step"=w523, "Previous Speed"=w525) -> ("New Speed"=w524:dbl)
          n294 = Bundle("New Speed"=w524, w527, w527, w527) -> (w528:cluster{"New Speed":dbl, dbl, dbl, dbl})  [unwired: 1 in]
        }
      }
    }
    frame "A" {
      # "Switch-case to determine which the second button is."
      n295 = case shown="\"W\"" w531 {
        tunnel: [w542 w553 w564 w575 w585 w596 w599 w608] -> w530
        tunnel: w532 -> [w533 w545 w555 w565 w577 w589 _ w601]
        tunnel: w529 -> [w541 w550 w562 w568 w583 w592 _ w605]
        frame "UP" {
          w538 = 0.0
          n296 = Unbundle(w541) -> ("Roll"=w535:sgl, "Yaw Speed"=w534:sgl)  [unwired: 2 out]
          n297 = call "Speed Calculator.vi"("Speed step"=w533, "Previous Speed"=w534) -> ("New Speed"=w536:dbl)
          n298 = Absolute Value(x=w535) -> (abs(x)=w540:sgl)
          n299 = call "Speed Calculator.vi"("Speed step"=w533, "Previous Speed"=w540) -> ("New Speed"=w539:dbl)
          n300 = Negate(x=w539) -> (-x=w537:dbl)
          n301 = Bundle(w537, w538, "New Speed"=w536, w538) -> (w542:cluster{dbl, dbl, "New Speed":dbl, dbl})  [unwired: 1 in]
        }
        frame "DOWN" {
          w554 = 0.0
          n302 = Unbundle(w550) -> ("Pitch"=w549:sgl, "Vertical Speed"=w548:sgl)  [unwired: 2 out]
          n303 = Absolute Value(x=w549) -> (abs(x)=w546:sgl)
          n304 = Absolute Value(x=w548) -> (abs(x)=w547:sgl)
          n305 = call "Speed Calculator.vi"("Speed step"=w545, "Previous Speed"=w546) -> ("New Speed"=w543:dbl)
          n306 = call "Speed Calculator.vi"("Speed step"=w545, "Previous Speed"=w547) -> ("New Speed"=w544:dbl)
          n307 = Negate(x=w543) -> (-x=w552:dbl)
          n308 = Negate(x=w544) -> (-x=w551:dbl)
          n309 = Bundle(w554, w552, w551, w554) -> (w553:cluster{dbl, dbl, dbl, dbl})  [unwired: 1 in]
        }
        frame "RIGHT" {
          w557 = 0.0
          n310 = Unbundle(w562) -> ("Roll"=w561:sgl, "Yaw Speed"=w556:sgl)  [unwired: 2 out]
          n311 = call "Speed Calculator.vi"("Speed step"=w555, "Previous Speed"=w556) -> ("New Speed"=w558:dbl)
          n312 = Absolute Value(x=w561) -> (abs(x)=w560:sgl)
          n313 = call "Speed Calculator.vi"("Speed step"=w555, "Previous Speed"=w560) -> ("New Speed"=w559:dbl)
          n314 = Negate(x=w559) -> (-x=w563:dbl)
          n315 = Bundle(w563, w557, w557, "New Speed"=w558) -> (w564:cluster{dbl, dbl, dbl, "New Speed":dbl})  [unwired: 1 in]
        }
        frame "LEFT" {
          w574 = 0.0
          n316 = Unbundle(w568) -> ("Roll"=w567:sgl, "Yaw Speed"=w566:sgl)  [unwired: 2 out]
          n317 = Absolute Value(x=w567) -> (abs(x)=w570:sgl)
          n318 = Absolute Value(x=w566) -> (abs(x)=w569:sgl)
          n319 = call "Speed Calculator.vi"("Speed step"=w565, "Previous Speed"=w570) -> ("New Speed"=w572:dbl)
          n320 = call "Speed Calculator.vi"("Speed step"=w565, "Previous Speed"=w569) -> ("New Speed"=w571:dbl)
          n321 = Negate(x=w572) -> (-x=w573:dbl)
          n322 = Negate(x=w571) -> (-x=w576:dbl)
          n323 = Bundle(w573, w574, w574, w576) -> (w575:cluster{dbl, dbl, dbl, dbl})  [unwired: 1 in]
        }
        frame "S" {
          w586 = 0.0
          n324 = Unbundle(w583) -> ("Roll"=w582:sgl, "Pitch"=w579:sgl)  [unwired: 2 out]
          n325 = call "Speed Calculator.vi"("Speed step"=w577, "Previous Speed"=w579) -> ("New Speed"=w578:dbl)
          n326 = Absolute Value(x=w582) -> (abs(x)=w581:sgl)
          n327 = call "Speed Calculator.vi"("Speed step"=w577, "Previous Speed"=w581) -> ("New Speed"=w580:dbl)
          n328 = Negate(x=w580) -> (-x=w584:dbl)
          n329 = Bundle(w584, "New Speed"=w578, w586, w586) -> (w585:cluster{dbl, "New Speed":dbl, dbl, dbl})  [unwired: 1 in]
        }
        frame "W" {
          w597 = 0.0
          n330 = Unbundle(w592) -> ("Roll"=w591:sgl, "Pitch"=w590:sgl)  [unwired: 2 out]
          n331 = Absolute Value(x=w591) -> (abs(x)=w594:sgl)
          n332 = Absolute Value(x=w590) -> (abs(x)=w593:sgl)
          n333 = call "Speed Calculator.vi"("Speed step"=w589, "Previous Speed"=w594) -> ("New Speed"=w587:dbl)
          n334 = call "Speed Calculator.vi"("Speed step"=w589, "Previous Speed"=w593) -> ("New Speed"=w588:dbl)
          n335 = Negate(x=w587) -> (-x=w598:dbl)
          n336 = Negate(x=w588) -> (-x=w595:dbl)
          n337 = Bundle(w598, w595, w597, w597) -> (w596:cluster{dbl, dbl, dbl, dbl})  [unwired: 1 in]
        }
        frame "D" {
          w600 = 0.0
          n338 = Bundle(w600, w600, w600, w600) -> (w599:cluster{dbl, dbl, dbl, dbl})  [unwired: 1 in]
        }
        frame Default {
          w606 = 0.0
          n339 = Unbundle(w605) -> ("Roll"=w604:sgl)  [unwired: 3 out]
          n340 = Absolute Value(x=w604) -> (abs(x)=w603:sgl)
          n341 = call "Speed Calculator.vi"("Speed step"=w601, "Previous Speed"=w603) -> ("New Speed"=w602:dbl)
          n342 = Negate(x=w602) -> (-x=w607:dbl)
          n343 = Bundle(w607, w606, w606, w606) -> (w608:cluster{dbl, dbl, dbl, dbl})  [unwired: 1 in]
        }
      }
    }
    frame Default {
      w610 = 0.0
      n344 = Bundle(w610, w610, w610, w610) -> (w609:cluster{dbl, dbl, dbl, dbl})  [unwired: 1 in]
    }
  }
  "Control Cluster" <- w7
  n345 = Bundle By Name(cluster=T1 {"Hover"=FALSE, "Land/Take off"=FALSE, "button 3"=FALSE, "button 4"=FALSE} ("Buttons control 2"), "Hover"=w2, "Land/Take off"=w1) -> (→"Buttons control":T1)
